vi "Disconnect.vi"(8 "error in (no error)":errorcluster, 11 "PostgreSQL in":refnum<class "PostgreSQL.lvclass">) -> (0 "error out":errorcluster, 3 "PostgreSQL out":refnum<class "PostgreSQL.lvclass">)   [LabVIEW 2018, in "Database.lvlib" / "PostgreSQL.lvclass"]
uses:
  PostgreSQL.lvclass
  DatabaseBaseClass/DatabaseBaseClass.lvclass
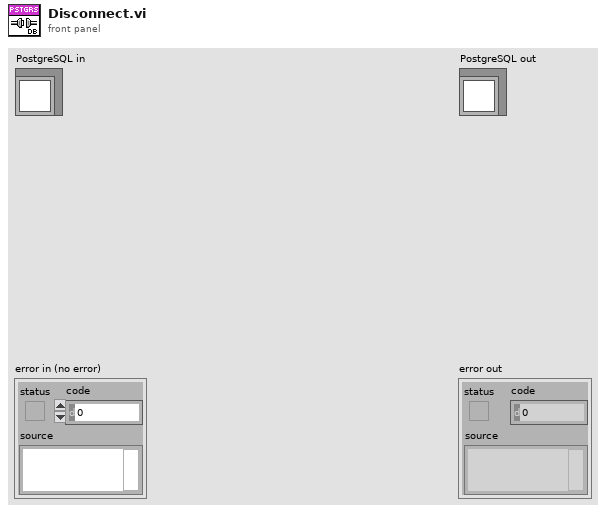
[diagram p1: front panel]
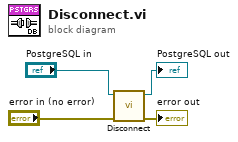
[diagram p0: block diagram]
diagram:
  n1 = call-parent "Disconnect.vi"("error in (no error)"="error in (no error)", "DatabaseBaseClass in"="PostgreSQL in") -> ("error out"=→"error out":errorcluster, "DatabaseBaseClass out"=→"PostgreSQL out":refnum<class "PostgreSQL.lvclass">)  [unwired: 8 in]
